vi "RSZVB Define Noise Figure Calibration Settings.vi"(4 "Port 2 (1)":i32=1, 5 "DUT Measurement Attenuation (0.0)":dbl format="%^.3e", 6 "Source Noise Cal Attenuation (0.0)":dbl format="%^.3e", 7 "External Attenuator (Off  (0)":bool, 8 "error in (no error)":errorcluster {"code" format="%.0x"}, 9 "Port 1 (1)":i32=1, 10 "Channel (1)":i32=1, 11 "VISA session":refnum<visa-resource-name>) -> (0 "error out":errorcluster {"code" format="%.0x"}, 3 "dup VISA session":refnum<visa-resource-name>)   [LabVIEW 2011]
doc: "This VI defines the calibration settings (port assignment, attenuations) for a noise figure calibration.\n\nNote(s):\n\n(1) This VI is available only with option R&S ZVAB-K30.\n\nRemote-control command(s):\n[SENSe<Ch>:]CORRection:COLLect:NFIGure:STARt"
uses:
  _utility/RSZVB Global Data.vi
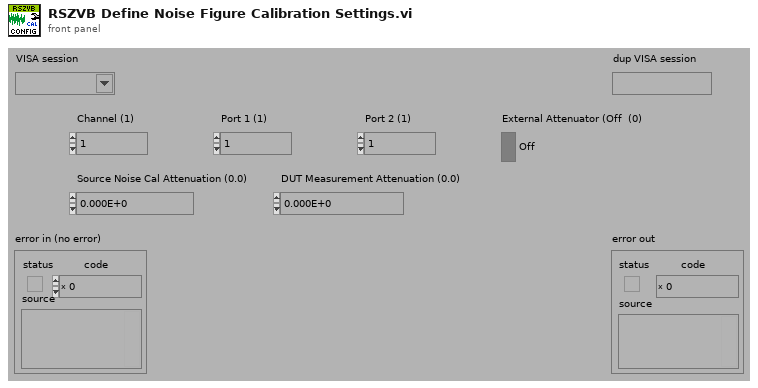
[diagram p1: front panel]
types:
  T1 = cluster{"Error Checking (T: On)":bool, "Installed Options":string[], "Data Valid?":bool, "Ports":i32, "Model":string[], "Option Checking (T: On)":bool}[]
  T2 = cluster{"Error Checking (T: On)":bool, "Installed Options":string[], "Data Valid?":bool, "Ports":i32, "Model":string[], "Option Checking (T: On)":bool}
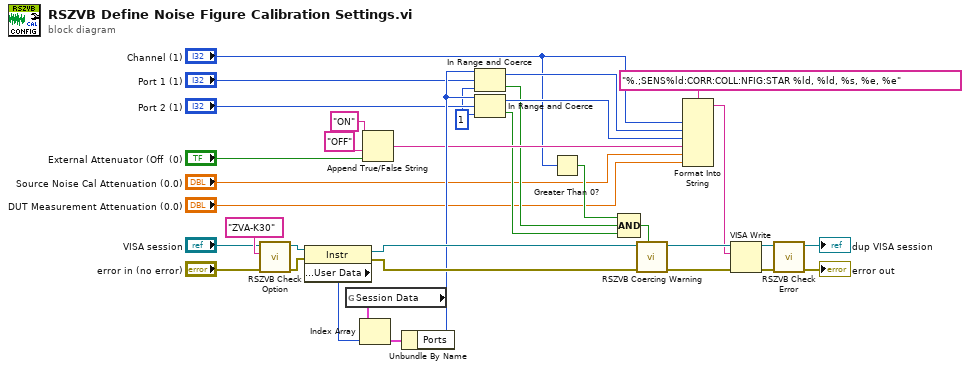
[diagram p0: block diagram]
diagram:
  w11 = 1 ("lower limit")
  n1 = call "RSZVB Check Option.vi"("error in (no error)"="error in (no error)", "Options"="ZVA-K30", "VISA session"="VISA session") -> ("error out"=w20:errorcluster, "dup VISA session"=w21:refnum<visa-resource-name>)  [unwired: 7 in]
  n2 = property class="Instr"(reference=w21, error in=w20) -> (reference out=w19:refnum<visa-resource-name>, error out=w18:errorcluster, "General Settings:User Data"=w24:u32)
  n3 = global read "RSZVB Global Data.vi" "Session Data"() -> (w23:T1)
  n4 = Index Array(array=w23, index=w24) -> (element=w22:T2)
  n5 = Append True/False String(1:"External Attenuator (Off  (0)", 2:"OFF" ("false string"), 3:"ON" ("true string")) -> (0:w10:string)  [unwired: 1 in]
  n6 = Unbundle By Name(w22) -> ("Ports"=w17:i32)
  n7 = In Range and Coerce(upper limit=w17, x="Port 1 (1)", lower limit=w11) -> (coerced(x)=w14:i32, In Range?=w8:bool)
  n8 = In Range and Coerce(upper limit=w17, x="Port 2 (1)", lower limit=w11) -> (coerced(x)=w13:i32, In Range?=w9:bool)
  n9 = Greater Than 0?(x="Channel (1)") -> (x > 0?=w7:bool)
  n10 = Compound Arithmetic op=AND(w7, w8, w9) -> (w5:bool)
  n11 = call "RSZVB Coercing Warning.vi"("In Range?"=w5, "error in (no error)"=w18, "VISA session"=w19) -> ("error out"=w29:errorcluster, "dup VISA session"=w30:refnum<visa-resource-name>)  [unwired: 7 in]
  n12 = Format Into String(format string="%.;SENS%ld:CORR:COLL:NFIG:STAR %ld, %ld, %s, %e, %e", "Channel (1)", w14, w13, w10, "Source Noise Cal Attenuation (0.0)", "DUT Measurement Attenuation (0.0)") -> (resulting string=w28:string)  [unwired: 2 in, 1 out]
  n13 = VISA Write(VISA resource name=w30, write buffer=w28, error in (no error)=w29) -> (VISA resource name out=w33:refnum<visa-resource-name>, error out=w32:errorcluster)  [unwired: 1 out]
  n14 = call "RSZVB Check Error.vi"("error in (no error)"=w32, "VISA session"=w33) -> ("error out"=→"error out":errorcluster, "dup VISA session"=→"dup VISA session":refnum<visa-resource-name>)  [unwired: 8 in]
